vi "util_launch_transition.vi"(5 "waitgroup":T3, 6 "recipe_data":variant, 7 "change_in_event":refnum<user-event>, 8 "error in (no error)":errorcluster, 9 "previous_state":T1, 10 "current_state":T1, 11 "transition_vi_reference":T2) -> (0 "error out":errorcluster)   [LabVIEW 2015, in "lv-recipe-machine.lvlib"]
uses:
  lv-recipe-machine.lvlib
  <userlib>/antonio-alexander/lv-waitgroup/public/_controls/api_waitgroup.ctl
  public/_controls/vi_reference_transition.ctl
  public/_controls/change.ctl
  public/_controls/automatic_state.ctl
  <userlib>/antonio-alexander/lv-waitgroup/lv-waitgroup.lvlib
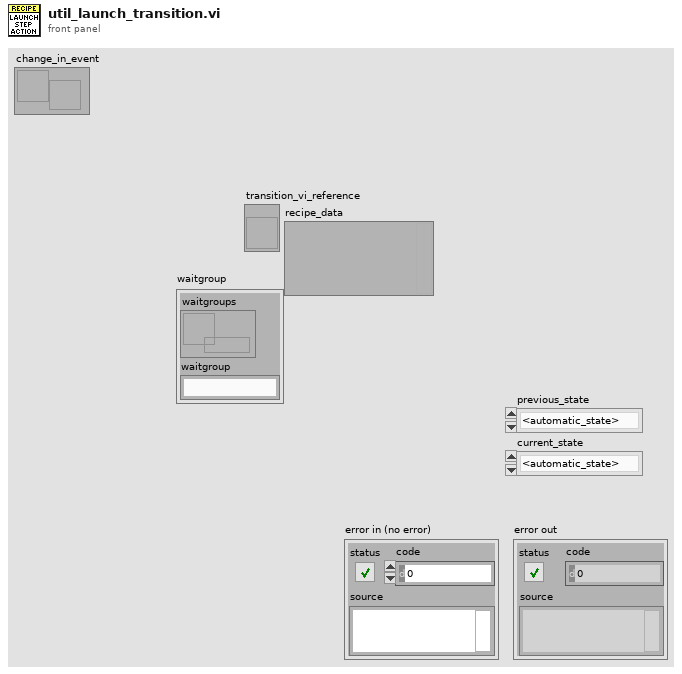
[diagram p1: front panel]
types:
  T1 = typedef "lv-recipe-machine.lvlib/automatic_state.ctl" = enum16{"<automatic_state>", "failed", "idle", "running", "paused", "transition", "stopped", "<null>"}
  T2 = typedef "lv-recipe-machine.lvlib/vi_reference_transition.ctl" = refnum<vi>
  T3 = typedef "lv-waitgroup.lvlib/api_waitgroup.ctl" = cluster{"waitgroups":refnum<data-value>, "waitgroup":string}
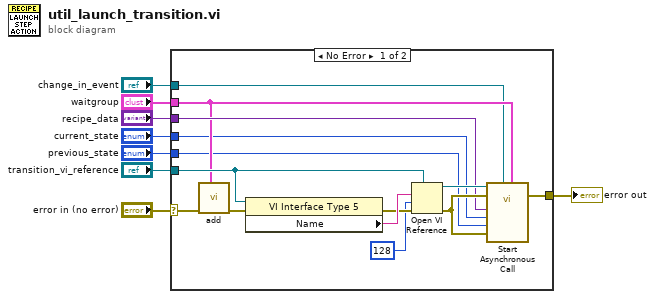
[diagram p0: block diagram]
diagram:
  n1 = case shown="No Error" "error in (no error)" {
    selector: "error in (no error)" -> [w16 w23]
    tunnel: "waitgroup" -> [w12 _]
    tunnel: [w15 w23] -> w6
    tunnel: "transition_vi_reference" -> [w14 _]
    tunnel: "recipe_data" -> [w13 _]
    tunnel: "change_in_event" -> [w11 _]
    tunnel: "current_state" -> [w10 _]
    tunnel: "previous_state" -> [w9 _]
    frame No Error {
      n2 = call <userlib>:"add.vi"("waitgroup"=w12, "error in (no error)"=w16) -> ("error out"=w21:errorcluster)  [unwired: 9 in]
      n3 = property class="VI Interface Type 5"(reference=w14, error in=w21) -> (error out=w19:errorcluster, "Name"=w20:string)  [unwired: 1 out]
      n4 = Open VI Reference(type specifier VI Refnum (for type only)=w14, vi path=w20, options=128, error in (no error)=w19) -> (vi reference=w18:T2, error out=w22:errorcluster)  [unwired: 2 in]
      n5 = call-by-ref "Start Asynchronous Call"(reference=w18, error in=w22, "waitgroup"=w12, "change_in_event"=w11, 8:"error in (no error)"=w22, "previous_state"=w9, "current_state"=w10, "recipe_data"=w13) -> (error out=w15:errorcluster)  [unwired: 5 in, 2 out]
    }
    frame Error {
    }
  }
  "error out" <- w6
